vi "Updater.vi"(8 "Error In":errorcluster, 10 "Waveform Chart":dynamicdata(graph), 11 "Display Panel.lvlib:Universal Display.lvclass":refnum<class "Universal Display.lvclass">) -> (0 "Error Out":errorcluster, 3 "Display Panel.lvlib:Universal Display.lvclass 2":refnum<class "Universal Display.lvclass">)   [LabVIEW 2014, in "Display Panel.lvlib" / "Universal Display.lvclass"]
uses:
  Universal Display.lvclass
  Universal Display.lvclass/Universal Display.ctl
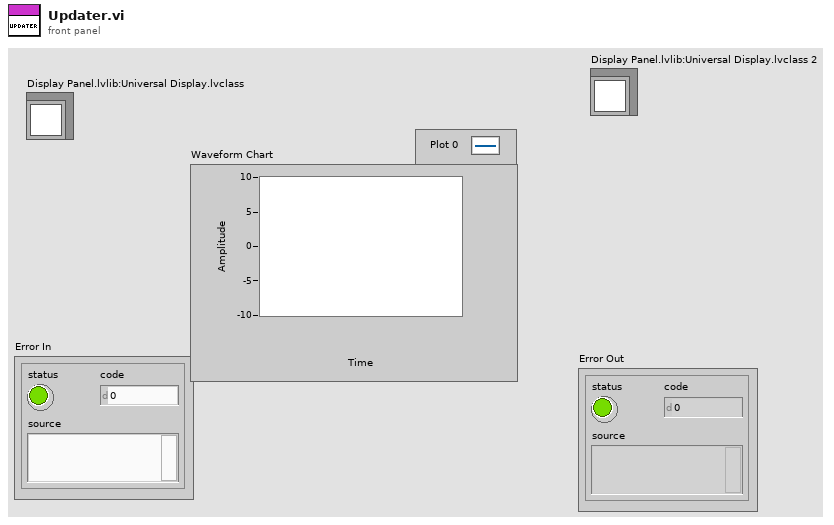
[diagram p1: front panel]
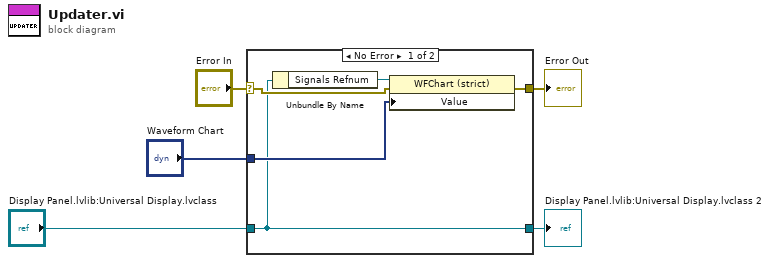
[diagram p0: block diagram]
diagram:
  n1 = case shown="No Error" "Error In" {
    selector: "Error In" -> [w8 w12]
    tunnel: "Display Panel.lvlib:Universal Display.lvclass" -> [w6 w11]
    tunnel: "Waveform Chart" -> [w9 _]
    tunnel: [w7 w12] -> w3
    tunnel: [w6 w11] -> w2
    frame No Error {
      n2 = Unbundle By Name(w6) -> ("Signals Refnum"=w10:refnum<vi>)
      n3 = property class="WFChart (strict)"(reference=w10, error in=w8, "Value"=w9) -> (error out=w7:errorcluster)  [unwired: 1 out]
    }
    frame Error {
    }
  }
  "Error Out" <- w3
  "Display Panel.lvlib:Universal Display.lvclass 2" <- w2
